vi "Copy Data to Mapped Notifier.vi"(11 "Variant":variant) -> ()   [LabVIEW 2023]
doc: "This VI looks at a data frame variant and sends it onto the notifier for that particular payload class and ID."
uses:
  Type Definitions/Data Frame.ctl
  Type Definitions/Data Frame Header.ctl
  Type Definitions/Payload Class.ctl
  Type Definitions/Device.ctl
  Type Definitions/Enum - Parameters.ctl
  Type Definitions/Enum - Metadata.ctl
  Type Definitions/Enumerated Constants/Software Monitor.ctl
  Type Definitions/Enum - Data.ctl
  Type Definitions/Enum - System State.ctl
  Type Definitions/Enum - Commands.ctl
  <userlib>/_OpenG.lib/lvdata/lvdata.llb/openg_variant.lvlib
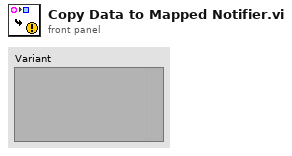
[diagram p1: front panel]
types:
  T1 = typedef "Data Frame.ctl" = cluster{"Frame Header":T2, "Payload":string, "CRC":u32}
  T2 = typedef "Data Frame Header.ctl" = cluster{"Sync":u32, "Time":dbl, "Nanosecond Counter":i64, "Payload Class":T3, "Payload ID":u16, "Counter":i32, "Options":u32, "Source":T4, "Destination":T4}
  T3 = typedef "Payload Class.ctl" = enum16{"System State", "Parameters", "Metadata", "Software Monitor", "Data", "Commands"}
  T4 = typedef "Device.ctl" = enum32{"None", "Exec", "Aux1", "Aux2", "Aux3"}
  T5 = typedef "Enum - Commands.ctl" = enum16{"Null", "Analog Output Command", "Digital Output Command"}
  T6 = typedef "Enum - Parameters.ctl" = enum16{"Device Parameters"}
  T7 = typedef "Enum - Metadata.ctl" = enum16{"Computer Metadata", "Computer Resources", "RT Image Metadata", "Startup Settings", "Telemetry Recorder Status"}
  T8 = typedef "Software Monitor.ctl" = enum16{"Internet Connection Monitor", "CPU Monitor", "Archive Monitor", "Memory Monitor", "Queue Monitor", "RTOS Update", "RTOS Monitor"}
  T9 = typedef "Enum - Data.ctl" = enum16{"Analog Input Data", "Notification Data", "Analog Output Data", "Digital Output Data", "Command Ack", "Digital Input Data", "GPS Solution Data"}
  T10 = typedef "Enum - System State.ctl" = enum16{"System Time", "Telemetry TCP State", "Writeable Drive State", "Command TCP State", "Network Adapter State", "Discovery Engine State", "Disk State"}
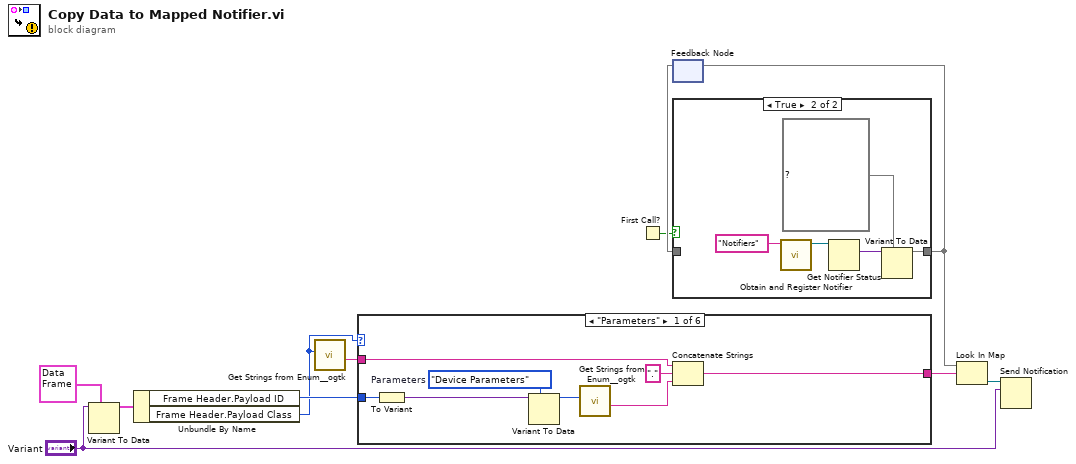
[diagram p0: block diagram]
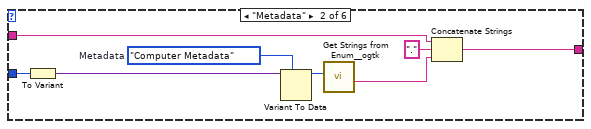
[diagram p3: hidden frame]
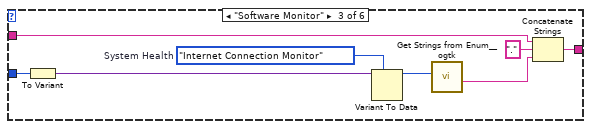
[diagram p4: hidden frame]
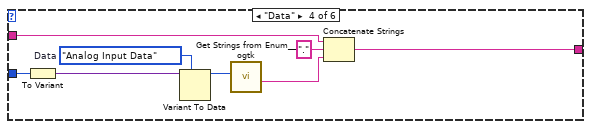
[diagram p5: hidden frame]
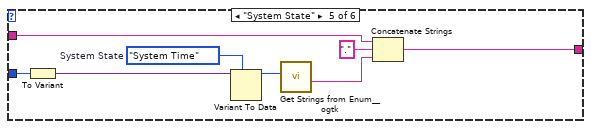
[diagram p6: hidden frame]
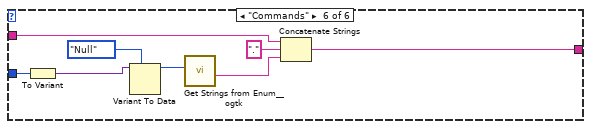
[diagram p7: hidden frame]
diagram:
  n1 = Variant To Data(type=T1 {"Frame Header"={"Sync"=0, "Time"=0.0, "Nanosecond Counter"=0, "Payload Class"=enum."System State", "Payload ID"=0, "Counter"=0, "Options"=0, "Source"=enum."None", "Destination"=enum."None"}, "Payload"="", "CRC"=0} ("Frame"), Variant="Variant") -> (data=w2:T1)  [unwired: 1 in, 1 out]
  n2 = Unbundle By Name(w2) -> ("Frame Header.Payload ID"=w4:u16, "Frame Header.Payload Class"=w3:T3)
  n3 = call <userlib>:"Get Strings from Enum__ogtk.vi"("Enum"=w3) -> ("String Value"=w5:string)  [unwired: 7 in, 3 out]
  n4 = case shown="\"Parameters\"" w3 {
    tunnel: w4 -> [w18 w26 w34 w42 w50 w58]
    tunnel: w5 -> [w15 w24 w32 w40 w48 w56]
    tunnel: [w12 w21 w29 w37 w45 w53] -> w9
    frame "Parameters" {
      w17 = Enum_-_Parameters."Device Parameters"  # Parameters
      n5 = To Variant(anything=w18) -> (Variant=w19:variant)
      n6 = Variant To Data(type=w17, Variant=w19) -> (data=w16:T6)  [unwired: 1 in, 1 out]
      n7 = call <userlib>:"Get Strings from Enum__ogtk.vi"("Enum"=w16) -> ("String Value"=w13:string)  [unwired: 7 in, 3 out]
      n8 = Concatenate Strings(w15, "." ("string"), w13) -> (w12:string)
    }
    frame "Metadata" {
      w20 = Enum_-_Metadata."Computer Metadata"  # Metadata
      n9 = To Variant(anything=w26) -> (Variant=w27:variant)
      n10 = Variant To Data(type=w20, Variant=w27) -> (data=w25:T7)  [unwired: 1 in, 1 out]
      n11 = call <userlib>:"Get Strings from Enum__ogtk.vi"("Enum"=w25) -> ("String Value"=w22:string)  [unwired: 7 in, 3 out]
      n12 = Concatenate Strings(w24, "." ("string"), w22) -> (w21:string)
    }
    frame "Software Monitor" {
      w28 = Software_Monitor."Internet Connection Monitor"  # System Health
      n13 = To Variant(anything=w34) -> (Variant=w35:variant)
      n14 = Variant To Data(type=w28, Variant=w35) -> (data=w33:T8)  [unwired: 1 in, 1 out]
      n15 = call <userlib>:"Get Strings from Enum__ogtk.vi"("Enum"=w33) -> ("String Value"=w30:string)  [unwired: 7 in, 3 out]
      n16 = Concatenate Strings(w32, "." ("string"), w30) -> (w29:string)
    }
    frame "Data" {
      w36 = Enum_-_Data."Analog Input Data"  # Data
      n17 = To Variant(anything=w42) -> (Variant=w43:variant)
      n18 = Variant To Data(type=w36, Variant=w43) -> (data=w41:T9)  [unwired: 1 in, 1 out]
      n19 = call <userlib>:"Get Strings from Enum__ogtk.vi"("Enum"=w41) -> ("String Value"=w38:string)  [unwired: 7 in, 3 out]
      n20 = Concatenate Strings(w40, "." ("string"), w38) -> (w37:string)
    }
    frame "System State" {
      w44 = Enum_-_System_State."System Time"  # System State
      n21 = To Variant(anything=w50) -> (Variant=w51:variant)
      n22 = Variant To Data(type=w44, Variant=w51) -> (data=w49:T10)  [unwired: 1 in, 1 out]
      n23 = call <userlib>:"Get Strings from Enum__ogtk.vi"("Enum"=w49) -> ("String Value"=w46:string)  [unwired: 7 in, 3 out]
      n24 = Concatenate Strings(w48, "." ("string"), w46) -> (w45:string)
    }
    frame "Commands" {
      n25 = To Variant(anything=w58) -> (Variant=w59:variant)
      n26 = Variant To Data(type=Enum_-_Commands."Null" ("System State"), Variant=w59) -> (data=w57:T5)  [unwired: 1 in, 1 out]
      n27 = call <userlib>:"Get Strings from Enum__ogtk.vi"("Enum"=w57) -> ("String Value"=w54:string)  [unwired: 7 in, 3 out]
      n28 = Concatenate Strings(w56, "." ("string"), w54) -> (w53:string)
    }
  }
  n29 = First Call?() -> (First Call?: T/F=w6:bool)
  n30 = feedback #1() -> (w7:map{string, refnum<notifier>})  [unwired: 1 in]
  n31 = case shown="True" w6 {
    tunnel: [w60 w61] -> w8
    tunnel: w7 -> [w60 _]
    frame False {
    }
    frame True {
      n32 = call "Obtain and Register Notifier.vi"("name (unnamed)"="Notifiers") -> ("notifier out"=w63:refnum<notifier>)  [unwired: 8 in, 2 out]
      n33 = Get Notifier Status(notifier=w63) -> (current notification=w64:variant)  [unwired: 1 in, 4 out]
      n34 = Variant To Data(type=map{string, refnum<notifier>} {} ("map"), Variant=w64) -> (data=w61:map{string, refnum<notifier>})  [unwired: 1 in, 1 out]
    }
  }
  n35 = feedback-in #1(w8) -> ()
  n36 = Look In Map(map=w8, key=w9) -> (value=w10:refnum<notifier>)  [unwired: 1 in, 1 out]
  n37 = Send Notification(notification="Variant", notifier=w10) -> ()  [unwired: 1 in, 2 out]
